vi "Create All Message Queues.vi"(8 "error in (no error)":errorcluster) -> (0 "error out":errorcluster, 3 "Message Queues out":T1)   [LabVIEW 2021, in "Message Queue.lvlib"]
doc: "This VI creates and initializes all the message queues for your application. If your application requires more than one message queue, right-click the \"Message Queues\" constant above and select Open Type Def. Add the new Message Queue(s) to the type definition, then initialize them in this VI."
uses:
  Message Queue.lvlib
  All Message Queues.ctl
  Message Cluster.ctl
  Enqueue Message (Single).vi
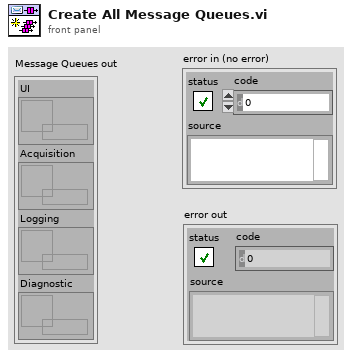
[diagram p1: front panel]
types:
  T1 = typedef "Message Queue.lvlib/All Message Queues.ctl" = cluster{"UI":refnum<queue>, "Acquisition":refnum<queue>, "Logging":refnum<queue>, "Diagnostic":refnum<queue>}
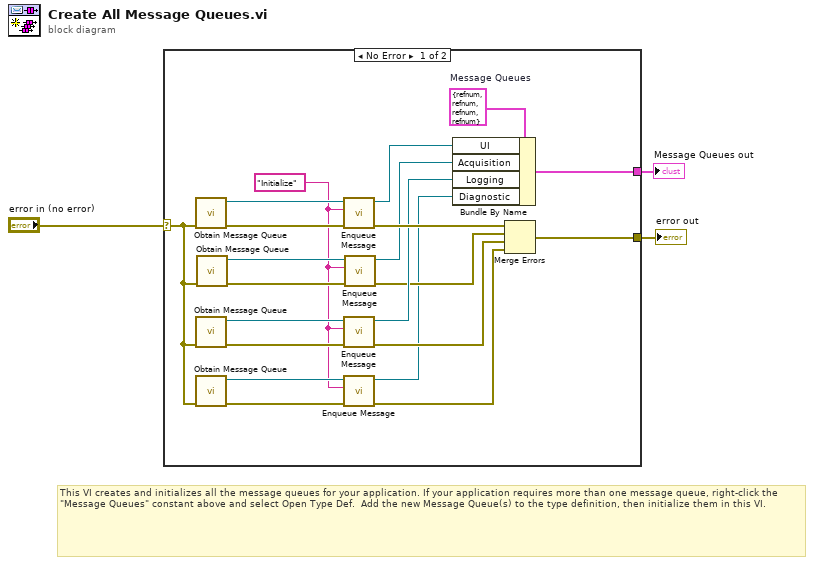
[diagram p0: block diagram]
diagram:
  # "This VI creates and initializes all the message queues for your application. If your application requires more than one message queue, right-click the \"Message Queues\" constant above and select Open Type Def.  Add the new Message Queue(s) to the type definition, then initialize them in this VI."
  n1 = case shown="No Error" "error in (no error)" {
    selector: "error in (no error)" -> [w9 w25]
    tunnel: [w12 w25] -> w3
    tunnel: [w22 _] -> w2
    frame No Error {
      w5 = "Initialize" ("Message")
      w23 = T1 {"UI"=refnum, "Acquisition"=refnum, "Logging"=refnum, "Diagnostic"=refnum}  # Message Queues
      n2 = call "Obtain Message Queue.vi"("error in (no error)"=w9) -> ("error out"=w21:errorcluster, "Message Queue"=w20:refnum<queue>)  [unwired: 9 in]
      n3 = call "Obtain Message Queue.vi"("error in (no error)"=w9) -> ("error out"=w17:errorcluster, "Message Queue"=w16:refnum<queue>)  [unwired: 9 in]
      n4 = call "Obtain Message Queue.vi"("error in (no error)"=w9) -> ("error out"=w8:errorcluster, "Message Queue"=w6:refnum<queue>)  [unwired: 9 in]
      n5 = call "Obtain Message Queue.vi"("error in (no error)"=w9) -> ("error out"=w18:errorcluster, "Message Queue"=w19:refnum<queue>)  [unwired: 9 in]
      n6 = call-poly "Enqueue Message.vi"("error in (no error)"=w21, "Message"=w5, "Message Queue"=w20) -> ("error out"=w24:errorcluster, "dup Message Queue"=w15:refnum<queue>)  [unwired: 7 in]
      n7 = call-poly "Enqueue Message.vi"("error in (no error)"=w17, "Message"=w5, "Message Queue"=w16) -> ("error out"=w10:errorcluster, "dup Message Queue"=w13:refnum<queue>)  [unwired: 7 in]
      n8 = call-poly "Enqueue Message.vi"("error in (no error)"=w8, "Message"=w5, "Message Queue"=w6) -> ("error out"=w7:errorcluster, "dup Message Queue"=w4:refnum<queue>)  [unwired: 7 in]
      n9 = call-poly "Enqueue Message.vi"("error in (no error)"=w18, "Message"=w5, "Message Queue"=w19) -> ("error out"=w11:errorcluster, "dup Message Queue"=w14:refnum<queue>)  [unwired: 7 in]
      n10 = Bundle By Name(cluster=w23, "UI"=w15, "Acquisition"=w14, "Logging"=w13, "Diagnostic"=w4) -> (w22:T1)
      n11 = Merge Errors(w24, w11, w10, w7) -> (w12:errorcluster)
    }
    frame Error {
    }
  }
  "Message Queues out" <- w2
  "error out" <- w3
